vi "GOMDBTS2048 get Color CIE170.vi"(0 "handle":i32, 11 "error in (no error)":errorcluster) -> (3 "Y_F":dbl, 4 "L_MB":dbl, 6 "M_MB":dbl, 8 "S_MB":dbl, 10 "X_F":dbl, 12 "function return":i32, 14 "Z_F":dbl, 15 "error out":errorcluster)   [LabVIEW 2015, in "GOMDBTS2048.lvlib"]
doc: "GOBTS2048DLL int __stdcall GOMDBTS2048_getColor(int handle, double* UpperX, double* UpperY, double* UpperZ, double* x, double* y,\n double* us, double* vs, double* CCT, double* domWL);"
uses:
  GOMDBTS2048.lvlib
  runtime/GOMDBTS2048.dll
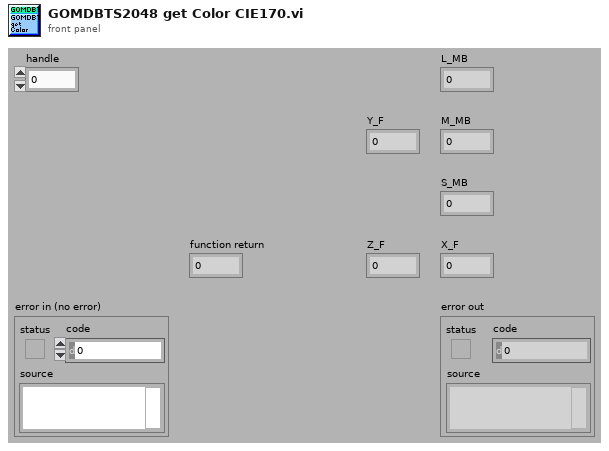
[diagram p1: front panel]
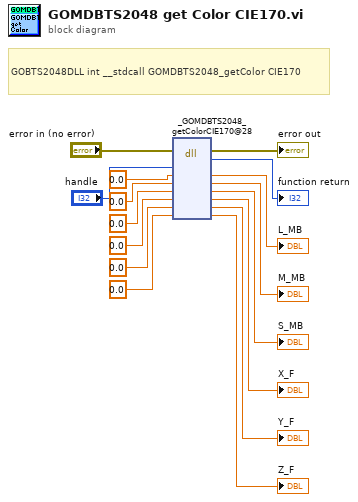
[diagram p0: block diagram]
diagram:
  # "GOBTS2048DLL int __stdcall GOMDBTS2048_getColor CIE170"
  n1 = dll-call lib="C:/Users/rkoch/Documents/GO_Library/runtime/GOMDBTS2048.*" fn="_GOMDBTS2048_getColorCIE170@28"(error in="error in (no error)", "handle"="handle", "L_MB"=0.0 ("UpperX"), "M_MB"=0.0 ("UpperY"), "S_MB"=0.0 ("UpperZ"), "X_F"=0.0 ("x"), "Y_F"=0.0 ("y"), "Z_F"=0.0 ("us")) -> (error out=→"error out":errorcluster, "return type"=→"function return":i32, "L_MB"=→"L_MB":dbl, "M_MB"=→"M_MB":dbl, "S_MB"=→"S_MB":dbl, "X_F"=→"X_F":dbl, "Y_F"=→"Y_F":dbl, "Z_F"=→"Z_F":dbl)  [unwired: 3 in, 1 out]
